vi "Get Deadband Offset.vi"() -> (3 "死区偏移":dbl)   [LabVIEW 2013, in "Cooler.lvlib" / "Cooler.lvclass"]
doc: "冷却器有一个设定的需要维持的温度。为防止实际温度与设定温度非常接近时，系统在打开和关闭状态之间快速切换，设置一个死区－实际温度在这个范围之内时，系统的开关状态保持不变。对于“冷却器”类，这个范围是固定的，用户无法调整。由本子VI返回这个范围常量。"
uses:
  Cooler.lvclass
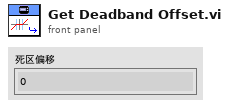
[diagram p1: front panel]
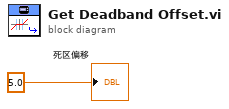
[diagram p0: block diagram]
diagram:
  "死区偏移" <- 5.0 ("y")
